vi "Confirm and Return Node Path.vi"(6 "Overwrite Existing?":bool, 8 "error in (no error)":errorcluster, 9 "New Node Path":string, 10 "Base Node Path":string, 11 "SysDef Ref":T1) -> (0 "error out":errorcluster, 2 "Node Ref":refnum<k24>, 3 "SysDef Ref Out":T1)   [LabVIEW 2019, in "Simple SysDef API.lvlib"]
uses:
  <userlib>/SimpleSysDef/Simple SysDef API.lvlib
  NationalInstruments.VeriStand.SystemDefinitionAPI
  <userlib>/SimpleSysDef/_SubVIs/System Definition Reference.ctl
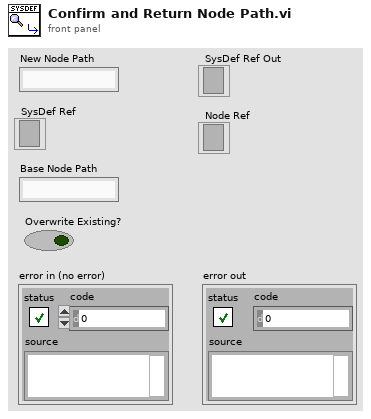
[diagram p1: front panel]
types:
  T1 = typedef "Simple SysDef API.lvlib/System Definition Reference.ctl" = refnum<k24>
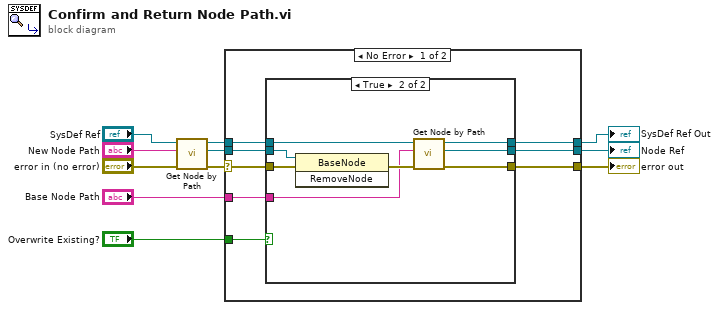
[diagram p0: block diagram]
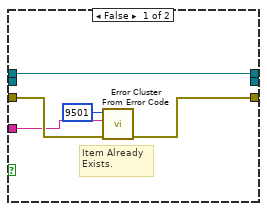
[diagram p2: hidden frame]
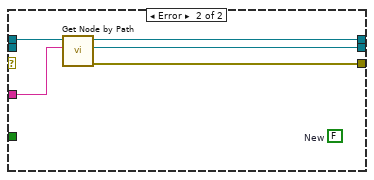
[diagram p3: hidden frame]
diagram:
  n1 = call <userlib>:"Get Node by Path.vi"("error in (no error)"="error in (no error)", "System Definition Node Path"="New Node Path", "SysDef Ref"="SysDef Ref") -> ("error out"=w7:errorcluster, "Node Ref"=w9:refnum<k24>, "SysDef Ref Out"=w8:T1)  [unwired: 6 in]
  n2 = case shown="No Error" w7 {
    selector: w7 -> [w19 _]
    tunnel: [w18 w37] -> w5
    tunnel: "Base Node Path" -> [w16 w36]
    tunnel: w8 -> [w13 w35]
    tunnel: [w12 w34] -> w3
    tunnel: [w14 w33] -> w4
    tunnel: w9 -> [w15 _]
    tunnel: "Overwrite Existing?" -> [w17 _]
    frame No Error {
      n3 = case shown="True" w17 {
        tunnel: w19 -> [w23 w31]
        tunnel: [w22 w29] -> w18
        tunnel: w16 -> [w21 w28]
        tunnel: w15 -> [_ w32]
        tunnel: [_ w27] -> w14
        tunnel: w13 -> [w20 w26]
        tunnel: [w20 w25] -> w12
        frame False {
          # "Item Already Exists."
          n4 = call <userlib>:"Error Cluster From Error Code.vi"("error in (no error)"=w23, "error message (\"\")"=w21, "error code (0)"=9501 ("code")) -> ("error out"=w22:errorcluster)  [unwired: 6 in]
        }
        frame True {
          n5 = invoke class="BaseNode" method="RemoveNode"(reference=w32, error in=w31) -> (error out=w30:errorcluster)  [unwired: 1 in, 2 out]
          n6 = call <userlib>:"Get Node by Path.vi"("error in (no error)"=w30, "System Definition Node Path"=w28, "SysDef Ref"=w26) -> ("error out"=w29:errorcluster, "Node Ref"=w27:refnum<k24>, "SysDef Ref Out"=w25:T1)  [unwired: 6 in]
        }
      }
    }
    frame Error {
      (unwired) FALSE  # New
      n7 = call <userlib>:"Get Node by Path.vi"("System Definition Node Path"=w36, "SysDef Ref"=w35) -> ("error out"=w37:errorcluster, "Node Ref"=w33:refnum<k24>, "SysDef Ref Out"=w34:T1)  [unwired: 7 in]
    }
  }
  "error out" <- w5
  "Node Ref" <- w4
  "SysDef Ref Out" <- w3
